vi "HowForebrainPerception.vi"(1 "How?MidbrainIn":cluster{"T":dbl, "Battey":dbl, "Temp":dbl}) -> (4 "BatteryGauge":dbl)   [LabVIEW 2010]
doc: "This SubVI takes clean How sense data from the Midbrain and layers perception onto it to be passed to the THINK processes in the Forebrain"
uses:
  6-OCU Neurons/CommonIndicators.ctl
  5.0-Global.vi
panel:
  # "This SubVI adds \nperception onto the\nHow data comming\nfrom the Midbrain"
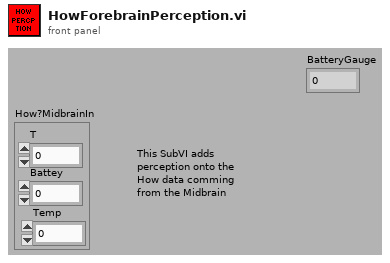
[diagram p1: front panel]
types:
  T1 = typedef "CommonIndicators.ctl" = cluster{"Speed":dbl, " Heading":cluster{dbl, dbl}, "MissionTime":dbl, "Battery":dbl, "MAP":bool, "LIDAR":bool, "ManualMissionMap":picture, "ManualModeLIDAR":picture, "ManualModeStop":bool, "How?":bool, "Where?":bool, "What?":bool, "ActManual":bool, "CollisionLight ":bool, "Ready":bool}
  T2 = cluster{"X (Current)":dbl, "Y (Current) ":dbl, "Heading":dbl, "Steering Angle":dbl}
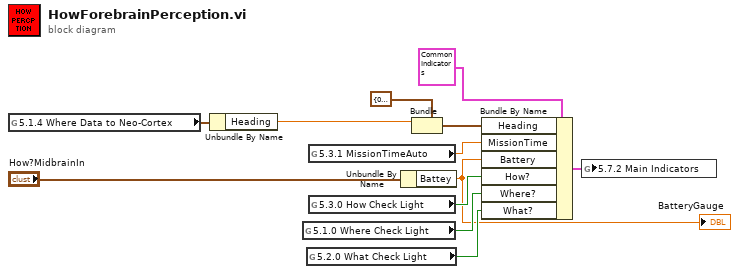
[diagram p0: block diagram]
diagram:
  n1 = global read "5.0-Global.vi" "5.1.4 Where Data to Neo-Cortex"() -> (w9:T2)
  n2 = Unbundle By Name(w9) -> ("Heading"=w6:dbl)
  n3 = global read "5.0-Global.vi" "5.1.0 Where Check Light"() -> (w2:bool)
  n4 = global read "5.0-Global.vi" "5.2.0 What Check Light"() -> (w3:bool)
  n5 = global read "5.0-Global.vi" "5.3.1 MissionTimeAuto"() -> (w5:dbl)
  n6 = global read "5.0-Global.vi" "5.3.0 How Check Light"() -> (w4:bool)
  n7 = Unbundle By Name("How?MidbrainIn") -> ("Battey"=w1:dbl)
  "BatteryGauge" <- w1
  n8 = Bundle(cluster=cluster{dbl, dbl} {0.0, 0.0} ("Heading"), w6) -> (w8:cluster{dbl, dbl})  [unwired: 1 in]
  n9 = Bundle By Name(cluster=T1 {"Speed"=0.0, " Heading"={0.0, 34.390870865624734}, "MissionTime"=0.0, "Battery"=0.0, "MAP"=FALSE, "LIDAR"=FALSE, "ManualMissionMap"=bytes[0], "ManualModeLIDAR"=bytes[0], "ManualModeStop"=FALSE, "How?"=FALSE, "Where?"=FALSE, "What?"=FALSE, "ActManual"=FALSE, "CollisionLight "=FALSE, "Ready"=FALSE} ("5.7.2 Main Indicators"), "Heading"=w8, "MissionTime"=w5, "Battery"=w1, "How?"=w4, "Where?"=w2, "What?"=w3) -> (w11:T1)
  n10 = global write "5.0-Global.vi" "5.7.2 Main Indicators"(w11) -> ()
